vi "Read Data.vi"(8 "error in (no error)":errorcluster, 11 "TX Speed in":refnum<class "TX Speed.lvclass">) -> (0 "error out":errorcluster, 3 "TX Speed out":refnum<class "TX Speed.lvclass">)   [LabVIEW 2020, in "TX Speed.lvclass"]
uses:
  TX Speed.lvclass
  TX Speed.lvclass/TX Speed.ctl
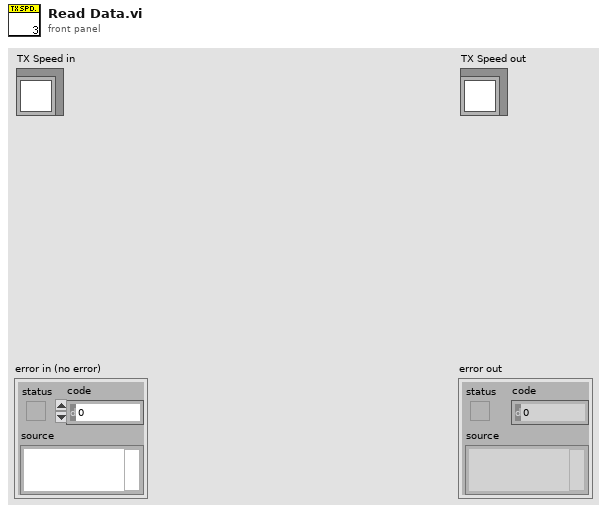
[diagram p1: front panel]
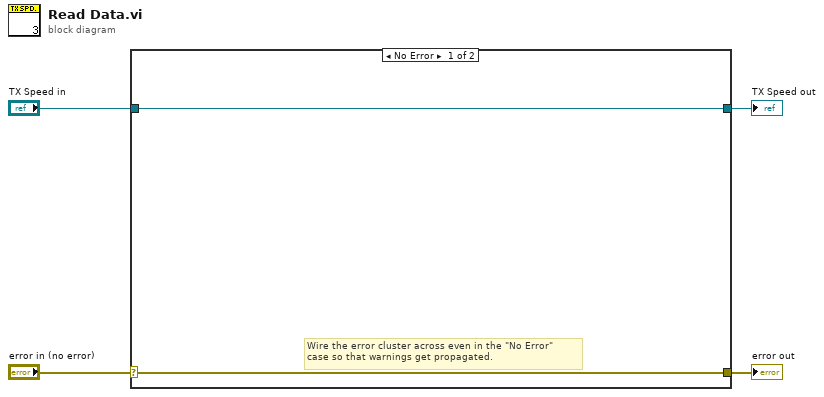
[diagram p0: block diagram]
diagram:
  n1 = case shown="No Error" "error in (no error)" {
    selector: "error in (no error)" -> [w5 w8]
    tunnel: [w5 w8] -> w3
    tunnel: [w6 w7] -> w1
    tunnel: "TX Speed in" -> [w6 w7]
    frame No Error {
      # "Wire the error cluster across even in the \"No Error\"\ncase so that warnings get propagated."
    }
    frame Error {
    }
  }
  "error out" <- w3
  "TX Speed out" <- w1
